vi "SetRef.vi"(8 "error in (no error)":errorcluster, 10 "Set External":bool, 11 "SigGen_ESG in":refnum<class "SigGen_ESG.lvclass">) -> (0 "error out":errorcluster, 3 "SigGen_ESG out":refnum<class "SigGen_ESG.lvclass">)   [LabVIEW 2014, in "SigGen_ESG.lvclass"]
uses:
  SigGen_ESG.lvclass
  SigGen_ESG.lvclass/SigGen_ESG.ctl
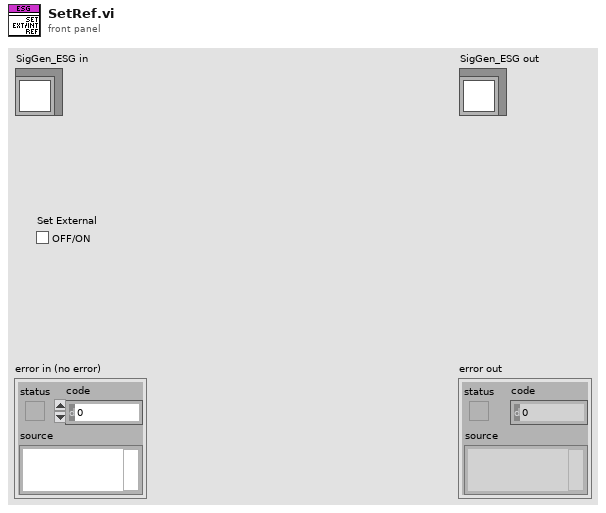
[diagram p1: front panel]
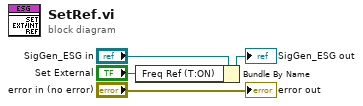
[diagram p0: block diagram]
diagram:
  n1 = Bundle By Name(cluster="SigGen_ESG in", "Freq Ref (T:ON)"="Set External") -> (→"SigGen_ESG out":refnum<class "SigGen_ESG.lvclass">)
  "error out" <- "error in (no error)"
